vi "Finish.vi"(8 "error in (no error)":errorcluster, 11 "Elevator Concrete in":refnum<class "Elevator Linear.lvclass">) -> (0 "error out":errorcluster, 3 "Elevator Concrete out":refnum<class "Elevator Linear.lvclass">)   [LabVIEW 2018, in "Elevator.lvlib" / "Elevator Linear.lvclass"]
uses:
  Elevator Linear.lvclass
  Elevator.lvclass
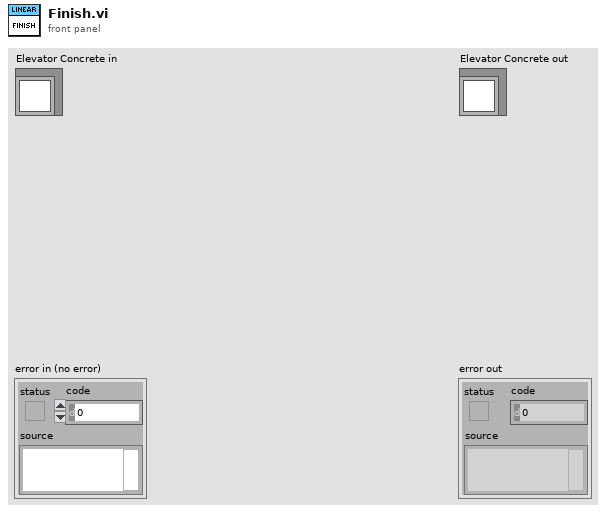
[diagram p1: front panel]
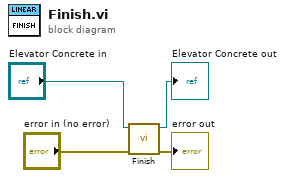
[diagram p0: block diagram]
diagram:
  n1 = call-parent "Finish.vi"("error in (no error)"="error in (no error)", "Elevator in"="Elevator Concrete in") -> ("error out"=→"error out":errorcluster, "Elevator out"=→"Elevator Concrete out":refnum<class "Elevator Linear.lvclass">)  [unwired: 8 in]
